vi "SOUR_POW_CORR_COLL_ACQ.vi"(0 "VISA IN":refnum<visa-resource-name>, 1 "Port number":i32, 2 "Power Meter Settings":string, 3 "Power Sensor":string, 4 "Source Port":string, 5 "error in":errorcluster, 7 "Channel":i32) -> (14 "VISA Out":refnum<visa-resource-name>, 19 "error out":errorcluster)   [LabVIEW 2018, in "PNA-X.lvlib"]
doc: "SOURce<cnum>:POWer<port>:CORRection:COLLect[:ACQuire] <char>,<id>[,src] \nNote: With PNA Rev. 6.2, a new \"id\" argument has been added to this command, replacing \nSOUR:POW:CORR:COLL:METH. \n(Write-only) Initiates a source power cal acquisition sweep using the power sensor attached to the \nspecified channel (A or B) on the power meter, or using the specified PNA receiver. \nNote: This command, when used with a power meter, cannot be sent over the GPIB unless the power \nmeter is connected to a different GPIB interface. Use one of the following methods to perform this \ncommand or its equivalent: \nIf present, use the GPIB dedicated controller port. \nConnect the power meter to the PNA using a USB / GPIB interface (Agilent 82357A). \nSCPI programming of the PNA using a LAN Client interface (see example) \nSend SCPI commands through the COM interface using the SCPI String Parser object. \nDirectly control the Power Meter and PNA to step frequency; then acquire and store the Power reading. \n(see example). \nParameters \n<cnum> Any existing channel number. If unspecified, value is set to 1 \n<port> Port number to correct for source power. If unspecified, value is set to 1. \n<char> The following choices are new beginning PNA Rev 6.2. Choose from: \nPMETer - Power Meter is used for all readings. \nPMReceiver - Power meter for the first iteration; then use the reference receiver \nfor remaining readings if necessary (same as \"fast iteration\" box checked on \n1835\n\ndialog box) \nRECeiver - Use PNA measurement receiver for all readings. \nThe following choices are superseded but still supported, in conjunction with \nSOUR:POW:CORR:COLL:METH. \nASENsor - Sensor on power meter channel A \nBSENsor - Sensor on power meter channel B \n<id> String. Not case sensitive. The power sensor or PNA receiver to use for \nmeasuring power. \nFor PMETer or PMRECeiver: select \"ASENSOR\" or \"BSENSOR\". \nFor RECeiver: select a PNA receiver to acquire readings using physical or logical \nreceiver notation. \nFor ASENsor or BSENsor, this argument is NOT required. \n[src] String. (NOT case sensitive). Source port. Optional. Use SOUR:CAT? to \nreturn a list of valid port names. \nWhile this argument can be used to make settings for ALL ports, it is designed \nto access ports that are not simple numbers, such as \"Port 1 Src2\". Otherwise, \nthe <port> argument performs the same function. If both arguments are \nspecified, [src] takes priority. \nExamples SOUR:POW:CORR:COLL PMET 'acquires power meter readings using \nthe A sensor. \nsource1:power2:correction:collect:acquire receiver,\"a1\" \n'acquires source cal readings using the reference receiver for \nport 1. \nQuery Syntax Not Applicable \nDefault Not Applicable \nSOURce:POWer:CORRection:COLLect:AVERage[:COUNt] <num> \n1836\n\n(Read-Write) This command, along with SOUR:POW:CORR:COLL:AVER:NTOLerance, allows for \nsettling of the power sensor READINGS. \nSpecifies the maximum number of power readings that are taken at each stimulus point to allow for \nmeasurement settling. Each reading is averaged with the previous readings at that stimulus point. \nWhen this average meets the Average:NTOLerance value or this number of readings has been made, \nthe average is returned as the valid reading. \nThis setting is not necessary when using a PNA receiver (SOUR:POW:CORR:COLL REC) to make \nthe measurement. \nLearn more. \nParameters \n<num> Maximum number of readings to make to allow for settling. Choose any \nnumber between 3 and 25. \nExamples SOUR:POW:CORR:COLL:AVER 2 \nsource:power:correction:collect:average:count 3 \nQuery Syntax SOURce:POWer:CORRection:COLLect:AVERage[:COUNt]? \nReturn Type Numeric \nDefault 3 \nSOURce:POWer:CORRection:COLLect:AVERage:NTOLerance <num> \n(Read-Write) This command, along with SOUR:POW:CORR:COLL:AVER:COUNT, allows for \nsettling of the power sensor READINGS. \nEach power reading is averaged with the previous readings at each stimulus point. When the average \nmeets this nominal tolerance value or the max number of readings has been made, the average is \nreturned as the valid reading. \nThis setting is not necessary when using a PNA receiver (SOUR:POW:CORR:COLL REC) to make \nthe measurement. \nLearn more. \nParameters \n<num> Power measurement settling tolerance value in dB. Choose any number \nbetween 0 and 5. \nExamples SOUR:POW:CORR:COLL:AVER:NTOL .05 \nsource1:power2:correction:collect:average:ntolerance .003 \n1837\n\nQuery Syntax SOURce:POWer:CORRection:COLLect:AVERage:NTOLerance? \nReturn Type Numeric \nDefault .050 dBm"
uses:
  PNA-X.lvlib
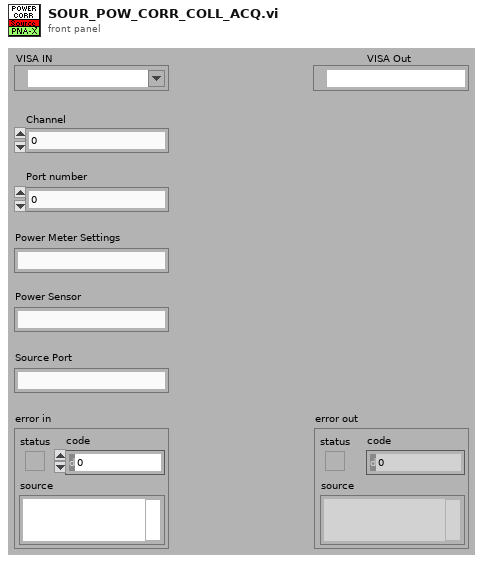
[diagram p1: front panel]
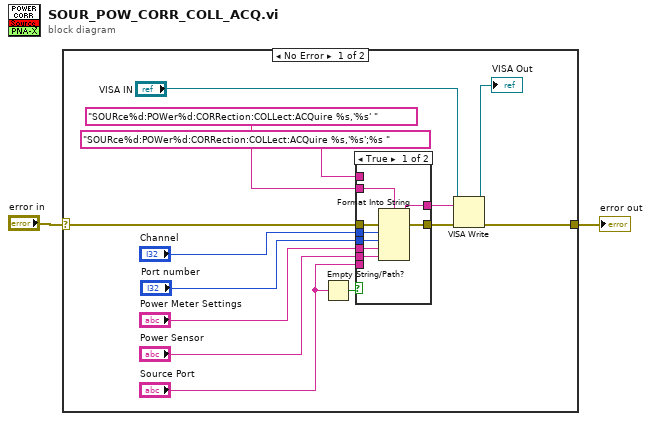
[diagram p0: block diagram]
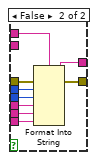
[diagram p2: hidden frame]
diagram:
  n1 = case shown="No Error" "error in" {
    selector: "error in" -> [w16 w34]
    tunnel: [w12 w34] -> w1
    frame No Error {
      n2 = Empty String/Path?(string/path="Source Port") -> (empty?=w6:bool)
      n3 = case shown="True" w6 {
        tunnel: w16 -> [w24 w33]
        tunnel: [w23 w32] -> w15
        tunnel: [w22 w31] -> w14
        tunnel: "Channel" -> [w21 w30]
        tunnel: "Port number" -> [w20 w29]
        tunnel: "Power Meter Settings" -> [w19 w28]
        tunnel: "Power Sensor" -> [w18 w27]
        tunnel: "Source Port" -> [_ w26]
        tunnel: "SOURce%d:POWer%d:CORRection:COLLect:ACQuire %s,'%s' " ("Cmdline") -> [w17 _]
        tunnel: "SOURce%d:POWer%d:CORRection:COLLect:ACQuire %s,'%s';%s " ("Cmdline") -> [_ w25]
        frame True {
          n4 = Format Into String(format string=w17, error in=w24, w21, w20, w19, w18) -> (resulting string=w22:string, error out=w23:errorcluster)  [unwired: 1 in]
        }
        frame False {
          n5 = Format Into String(format string=w25, error in=w33, w30, w29, w28, w27, w26) -> (resulting string=w31:string, error out=w32:errorcluster)  [unwired: 1 in]
        }
      }
      n6 = VISA Write(VISA resource name="VISA IN", write buffer=w14, error in (no error)=w15) -> (VISA resource name out=→"VISA Out":refnum<visa-resource-name>, error out=w12:errorcluster)  [unwired: 1 out]
    }
    frame Error {
    }
  }
  "error out" <- w1
